vi "DB_Execute Query.vi"(7 "Query":string="Select distinct", 8 "error in (no error)":errorcluster, 11 "connection reference":T1) -> (0 "error out":errorcluster, 3 "data":string[][](array[string]))   [LabVIEW 2017]
uses:
  <vilib>/addons/database/Connection.llb/Conn ObjectReference.ctl
  <vilib>/addons/database/Connection.llb/Conn Execute.vi
  <vilib>/addons/database/Recordset.llb/Rec Fetch Recordset Data (R).vi
  <vilib>/addons/database/Recordset.llb/Rec Destroy - Connection.vi
  <vilib>/addons/database/_DB Variant To Data/Database Variant To Data.xnode
  <vilib>/addons/database/NI_Database_API.lvlib
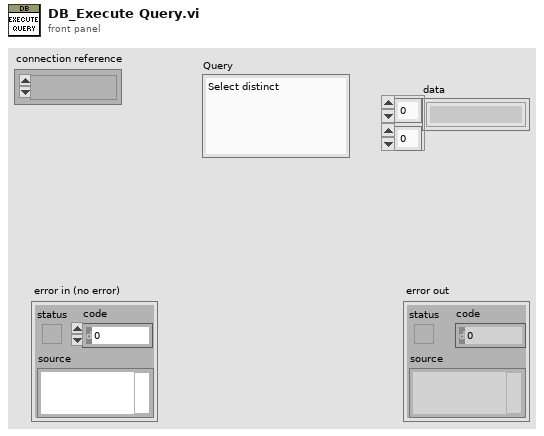
[diagram p1: front panel]
types:
  T1 = typedef "NI_Database_API.lvlib/Conn ObjectReference.ctl" = refnum<k1>
  T2 = typedef "NI_Database_API.lvlib/Rec ObjectReference.ctl" = refnum<k1>
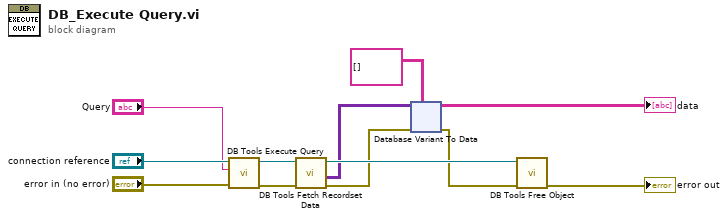
[diagram p0: block diagram]
diagram:
  n1 = call-poly <vilib>:"DB Tools Execute Query.vi"("error in (no error)"="error in (no error)", "SQL query"="Query", "connection reference"="connection reference") -> ("error out"=w8:errorcluster, "recordset reference"=w7:T2)  [unwired: 5 in]
  n2 = call-poly <vilib>:"DB Tools Fetch Recordset Data.vi"("error in (no error)"=w8, "recordset reference"=w7) -> ("error out"=w2:errorcluster, "recordset data"=w5:variant[][], "recordset reference out"=w6:T2)  [unwired: 3 in]
  n3 = xnode "Database Variant To Data"("database variant"=w5, "error in (no error)"=w2, "type"=string[][] [] ("format string")) -> ("data"=→"data":string[][], "error out"=w1:errorcluster)
  n4 = call-poly <vilib>:"DB Tools Free Object.vi"("error in (no error)"=w1, "recordset reference"=w6) -> ("error out"=→"error out":errorcluster)  [unwired: 8 in, 1 out]
